vi "UDCLaunchSettingsWindow.vi"(8 "Error In":errorcluster) -> (0 "Error Out":errorcluster)   [LabVIEW 2017, in "niceiplib.lvlib"]
doc: "UDC_SYMBOLS void UDCLaunchSettingsWindow();\n\nThis API is used to launch the CEIP settings application."
uses:
  <vilib>/UDC/niceiplib.lvlib
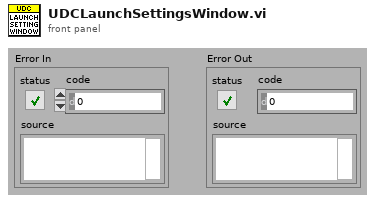
[diagram p1: front panel]
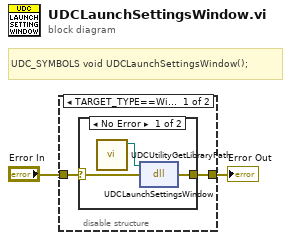
[diagram p0: block diagram]
diagram:
  # "UDC_SYMBOLS void UDCLaunchSettingsWindow();"
  n1 = disable-structure shown="TARGET_TYPE==Windows" {
    disable-tunnel: [w4 w9] -> w2
    disable-tunnel: "Error In" -> [w3 w9]
    frame condition #0 (active) {
      n2 = case shown="No Error" w3 {
        selector: w3 -> [w6 w8]
        tunnel: [w7 w8] -> w4
        frame No Error {
          n3 = call <vilib>:"UDCUtilityGetLibraryPath.vi"() -> ("Library Path"=w5:path)  [unwired: 11 in]
          n4 = dll-call lib="C:/2013LabVIEWCode/dist/vi.lib/UDC/niceiplib.*" fn="UDCLaunchSettingsWindow"(path in=w5, error in=w6) -> (error out=w7:errorcluster)  [unwired: 2 in, 1 out]
        }
        frame Error {
        }
      }
    }
    frame condition #1 {
    }
  }
  "Error Out" <- w2
